vi "Main.vi"(8 "error in":errorcluster, 11 "UserInterface in":refnum<class "UserInterface.lvclass">) -> (0 "error out":errorcluster, 3 "UserInterface out":refnum<class "UserInterface.lvclass">)   [LabVIEW 2021, in "UserInterface.lvclass"]
doc: "The Queued Message Handler of a Worker."
uses:
  UserInterface.lvclass
  C:/Program Files (x86)/National Instruments/LabVIEW 2021/vi.lib/addons/_Workers/Library/Classes/Worker/Worker.lvclass
  <vilib>/addons/_Workers/Library/Classes/Worker/Worker.lvclass/Worker.ctl
  UserInterface.lvclass/UserInterface.ctl
  WaveGenerator/WaveGenerator.lvclass
  Sine/Sine.lvclass
  C:/Users/chrismadlax/Desktop/LVSampleCode/WorkersComposite/Workers/WaveGenerator/WaveGenerator.lvclass
  Square/Square.lvclass
  Triangle/Triangle.lvclass
  <vilib>/addons/_Workers/Library/Classes/Message/Priority.ctl
  <vilib>/addons/_Workers/Library/Classes/Callback Message/Enqueue and Forget.vi
  <vilib>/addons/_Workers/Library/Classes/Message/Enqueue Message to Queue.vi
  <vilib>/addons/_Workers/Library/Classes/Callback Message/Enqueue and Collect.vi
  <vilib>/addons/_Workers/Library/Classes/Message/Enqueue Message to Self v2.vi
  Initialization Data.ctl
  <vilib>/addons/_Workers/Library/Classes/Worker/Worker.lvclass
  <vilib>/addons/_Workers/Library/Classes/Callback Message/Callback Message.lvclass
  <vilib>/addons/_Workers/Library/Classes/Message/Message.lvclass
  C:/Program Files (x86)/National Instruments/LabVIEW 2021/vi.lib/addons/_Workers/Library/Classes/Workers Object/Workers Object.lvclass
  C:/Users/chrismadlax/Desktop/LVSampleCode/WorkersComposite/Workers/UserInterface/UserInterface.lvclass
  <vilib>/addons/_Workers/Library/Classes/Message Queue/Message Queue.lvclass
panel:
  in  "StopM":bool
  out "ID":string
  in  "Destory":bool
  in  "Create":bool
  in  "Text Ring":enum16{"None", "Sine", "Square", "Triangle"}(ring)
  in  "Measure":bool
  out "W.Graph":waveform(dbl)(graph)
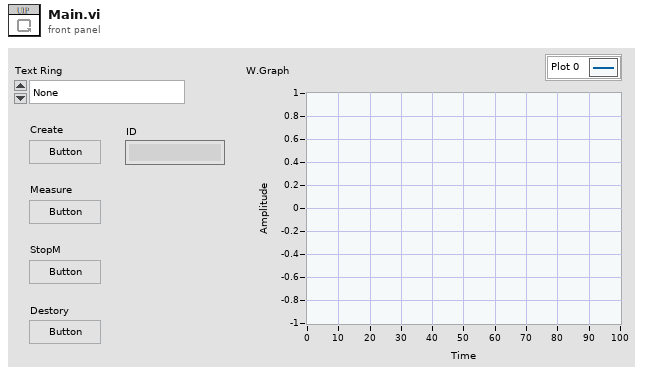
[diagram p1: front panel]
types:
  T1 = typedef "UserInterface.lvclass/Initialization Data.ctl" = cluster{"String":string}
  T2 = typedef "Workers.lvlib/Message.lvclass/Priority.ctl" = enum16{"Low", "Normal", "High"}
  T3 = typedef "Workers.lvlib/Case Label.ctl" = string
  T4 = cluster{"Message Queue out":refnum<class "Message Queue.lvclass">, "Case Label":T3}
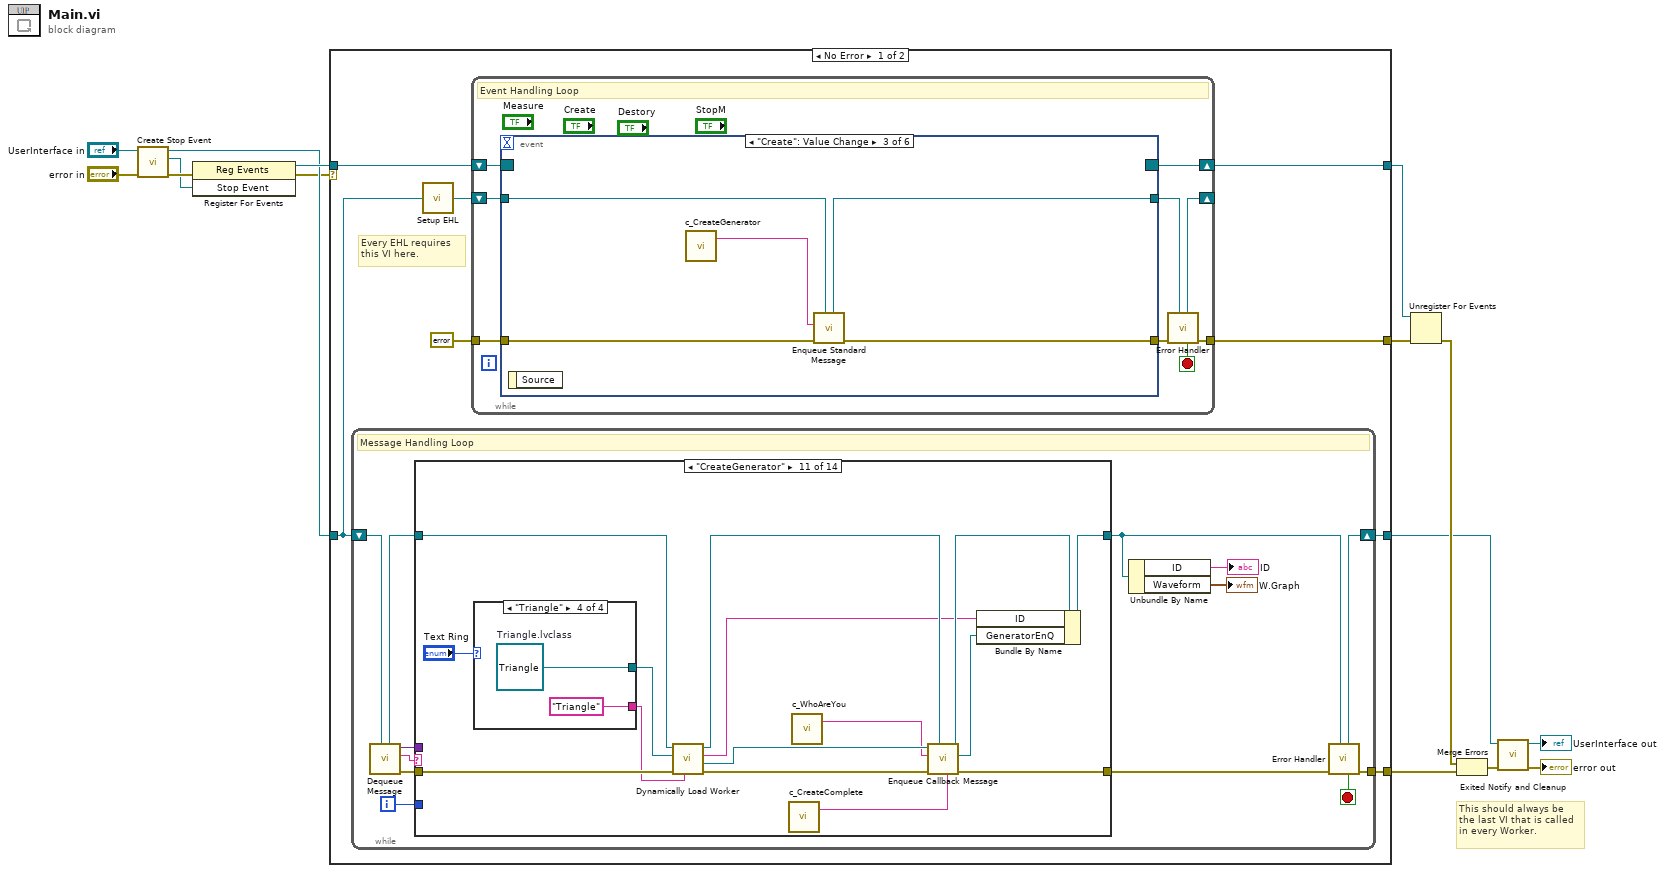
[diagram p0: block diagram]
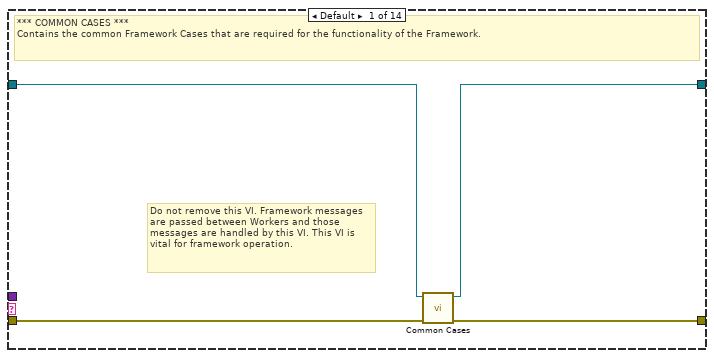
[diagram p2: hidden frame]
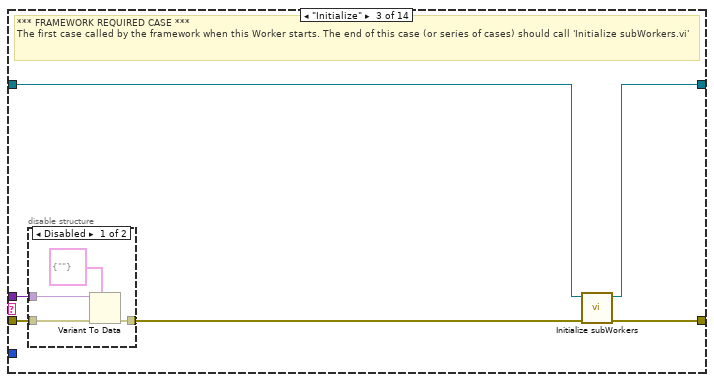
[diagram p4: hidden frame]
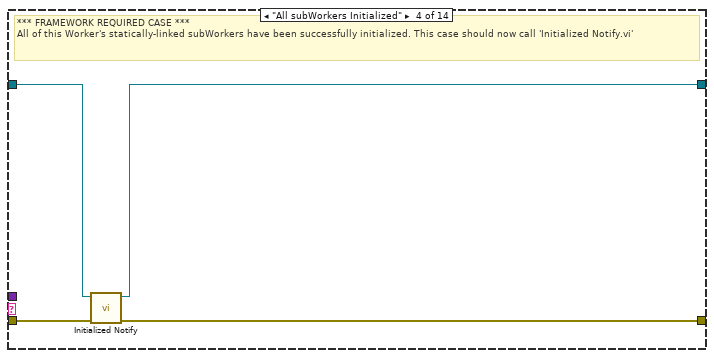
[diagram p6: hidden frame]
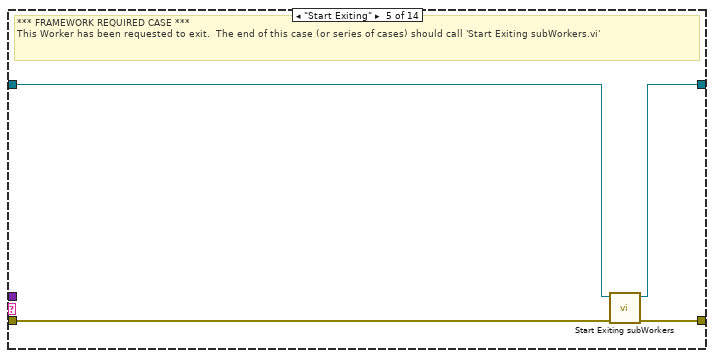
[diagram p7: hidden frame]
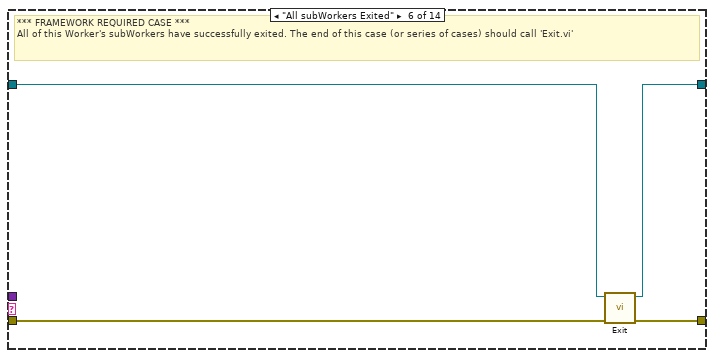
[diagram p8: hidden frame]
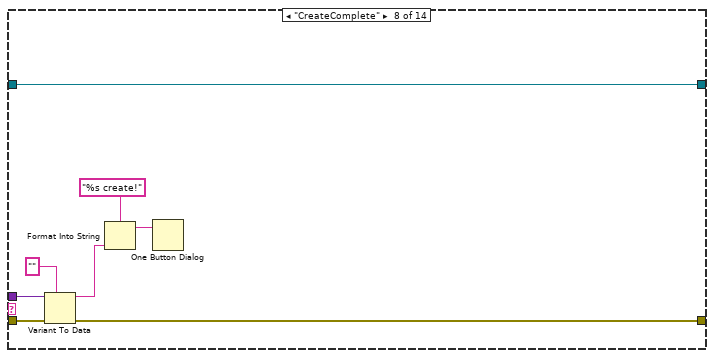
[diagram p10: hidden frame]
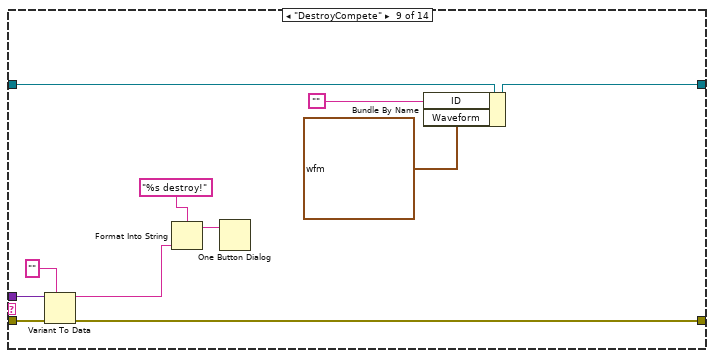
[diagram p11: hidden frame]
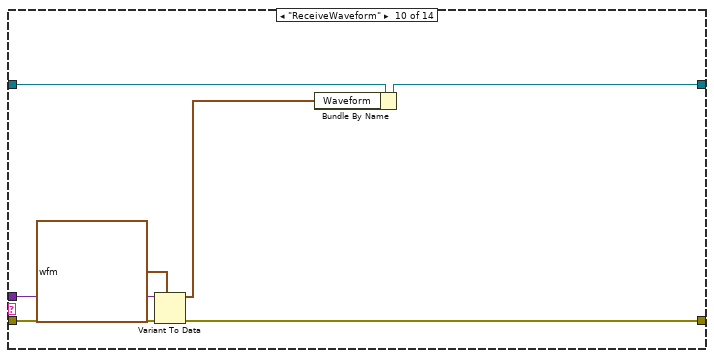
[diagram p12: hidden frame]
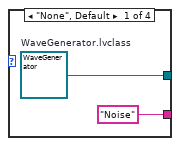
[diagram p13: hidden frame]
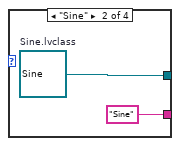
[diagram p14: hidden frame]
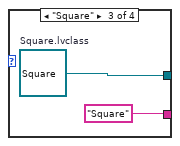
[diagram p15: hidden frame]
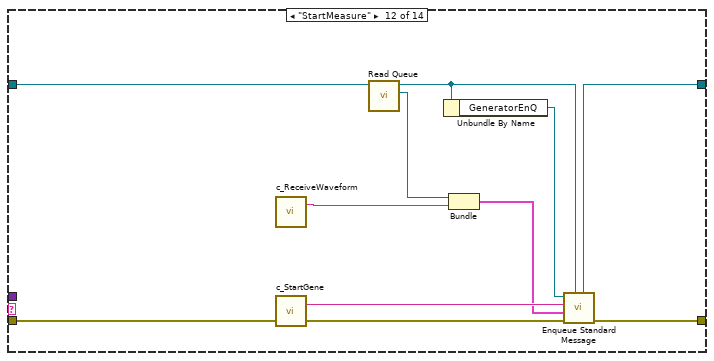
[diagram p16: hidden frame]
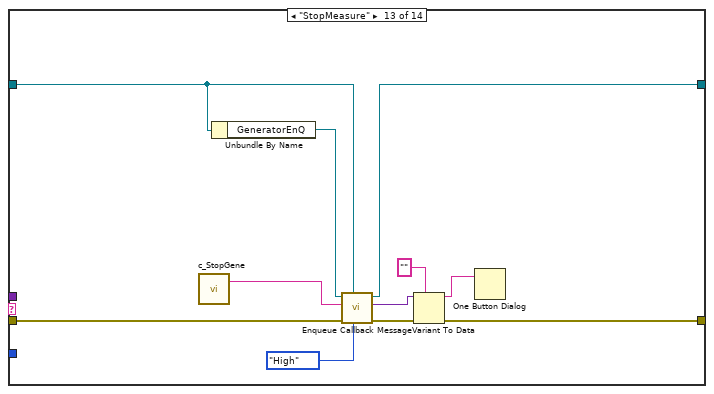
[diagram p17: hidden frame]
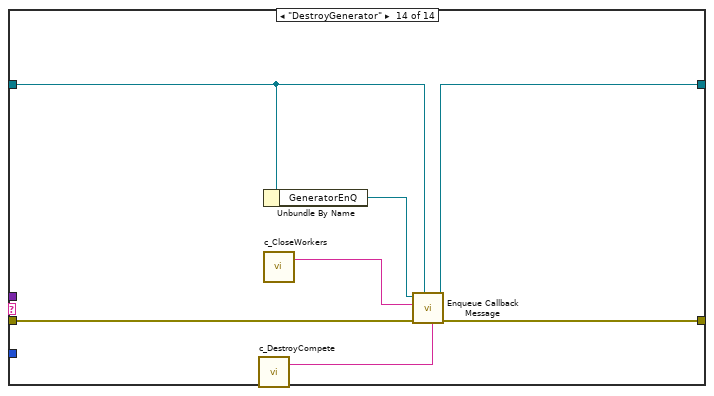
[diagram p18: hidden frame]
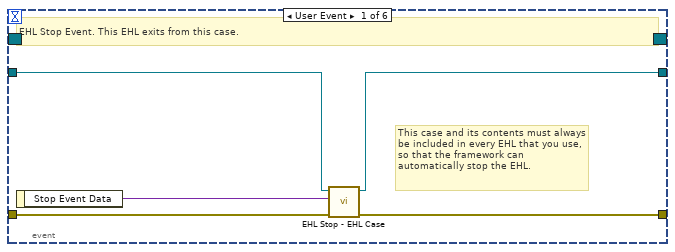
[diagram p19: hidden frame]
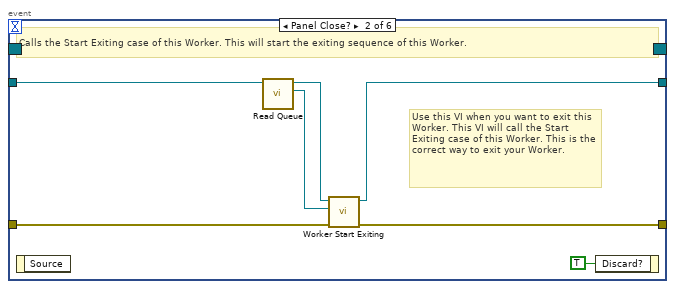
[diagram p20: hidden frame]
diagram:
  # "This should always be the last VI that is called in every Worker."
  n1 = call-dynamic "Create Stop Event.vi"("error in"="error in", "Worker"="UserInterface in") -> ("error out"=w10:errorcluster, "Stop Event"=w7:refnum<user-event>, "Worker out"=w4:refnum<class "UserInterface.lvclass">)  [unwired: 7 in]
  n2 = register-events(error in=w10, w7) -> (reference out=w9:refnum<event-registration>, error out=w2:errorcluster)  [unwired: 1 in]
  n3 = case shown="No Error" w2 {
    tunnel: w4 -> [w18 w187]
    tunnel: [w16 w188] -> w8
    tunnel: w9 -> [w23 w189]
    tunnel: [w20 w190] -> w14
    tunnel: [w22 w189] -> w13
    tunnel: [w17 w186] -> w11
    selector: w2 -> [_ w190]
    frame No Error {
      # "Every EHL requires\nthis VI here."
      n4 = while {
        shift-right: [w34] -> w17
        shift-left: w18 -> [w36]
        tunnel: [w35] -> w16
        i -> [w27]
        stop <- w28 stop-if-true
        # "Message Handling Loop"
        n5 = call-dynamic "Dequeue Message.vi"("Worker"=w36) -> ("error out"=w33:errorcluster, "Case out"=w29:string, "Data out"=w30:variant, "Worker out"=w31:refnum<class "UserInterface.lvclass">)  [unwired: 6 in, 1 out]
        n6 = case "Worker MHL Case Structure (DO NOT CHANGE LABEL NAME)" shown="\"CreateGenerator\"" w29 {
          tunnel: w33 -> [w40 w41 w46 w55 w58 w65 w66 w75 w86 w93 w108 w126 w137 w144]
          tunnel: [w39 w41 w48 w54 w61 w64 w66 w73 w84 w91 w101 w123 w130 w143] -> w32
          tunnel: w31 -> [w38 w42 w43 w57 w59 w63 w67 w74 w85 w92 w106 w125 w134 w141]
          tunnel: [w37 w42 w47 w56 w60 w62 w67 w74 w78 w88 w102 w122 w135 w142] -> w26
          tunnel: w30 -> [_ _ w44 _ _ _ _ w72 w83 w89 _ _ _ _]
          tunnel: w27 -> [_ _ _ _ _ _ _ _ _ _ _ _ _ _]
          frame Default {
            # "Do not remove this VI. Framework messages are passed between Workers and those messages are handled by this VI. This VI is vital for framework operation."
            # "*** COMMON CASES ***\nContains the common Framework Cases that are required for the functionality of the Framework."
            n7 = call-dynamic "Common Cases.vi"("error in"=w40, "Worker in"=w38) -> ("error out"=w39:errorcluster, "Worker out"=w37:refnum<class "UserInterface.lvclass">)  [unwired: 8 in]
          }
          frame "------ FRAMEWORK REQUIRED CASES ------" {
            # "Start of Framework Required Cases"
          }
          frame "Initialize" {
            # "*** FRAMEWORK REQUIRED CASE ***\nThe first case called by the framework when this Worker starts. The end of this case (or series of cases) should call 'Initialize subWorkers.vi'"
            n8 = disable-structure shown="Disabled" {
              disable-tunnel: w46 -> [w52 w53]
              disable-tunnel: [w51 w53] -> w45
              disable-tunnel: w44 -> [w50 _]
              frame Disabled {
                n9 = Variant To Data(error in=w52, type=T1 {"String"=""} ("Initialization Data"), Variant=w50) -> (error out=w51:errorcluster)  [unwired: 1 out]
              }
              frame Enabled {
              }
            }
            n10 = call-dynamic "Initialize subWorkers.vi"("error in"=w45, "Worker"=w43) -> ("error out"=w48:errorcluster, "dup Worker out"=w47:refnum<class "UserInterface.lvclass">)  [unwired: 8 in]
          }
          frame "All subWorkers Initialized" {
            # "*** FRAMEWORK REQUIRED CASE ***\nAll of this Worker's statically-linked subWorkers have been successfully initialized. This case should now call 'Initialized Notify.vi'"
            n11 = call-dynamic "Initialized Notify.vi"("error in"=w55, "Worker"=w57) -> ("error out"=w54:errorcluster, "dup Worker out"=w56:refnum<class "UserInterface.lvclass">)  [unwired: 8 in]
          }
          frame "Start Exiting" {
            # "*** FRAMEWORK REQUIRED CASE ***\nThis Worker has been requested to exit.  The end of this case (or series of cases) should call 'Start Exiting subWorkers.vi'"
            n12 = call-dynamic "Start Exiting subWorkers.vi"("error_in"=w58, "Worker"=w59) -> ("error out"=w61:errorcluster, "dup Worker out"=w60:refnum<class "UserInterface.lvclass">)  [unwired: 8 in]
          }
          frame "All subWorkers Exited" {
            # "*** FRAMEWORK REQUIRED CASE ***\nAll of this Worker's subWorkers have successfully exited. The end of this case (or series of cases) should call 'Exit.vi'"
            n13 = call-dynamic "Exit.vi"("error_in"=w65, "Worker"=w63) -> ("error out"=w64:errorcluster, "dup Worker out"=w62:refnum<class "UserInterface.lvclass">)  [unwired: 8 in]
          }
          frame "-----------------------------------------------" {
            # "End of Framework Required Cases"
          }
          frame "CreateComplete" {
            n14 = Variant To Data(error in=w75, type="", Variant=w72) -> (data=w69:string, error out=w73:errorcluster)
            n15 = Format Into String(format string="%s create!", w69) -> (resulting string=w68:string)  [unwired: 2 in, 1 out]
            n16 = One Button Dialog(message=w68) -> ()  [unwired: 1 in, 1 out]
          }
          frame "DestroyCompete" {
            n17 = Variant To Data(error in=w86, type="", Variant=w83) -> (data=w80:string, error out=w84:errorcluster)
            n18 = Format Into String(format string="%s destroy!", w80) -> (resulting string=w79:string)  [unwired: 2 in, 1 out]
            n19 = One Button Dialog(message=w79) -> ()  [unwired: 1 in, 1 out]
            n20 = Bundle By Name(cluster=w85, "ID"="", "Waveform"=waveform(dbl) {"t0"=timestamp(0 s since 1904-01-01), "dt"=1.0, "Y"=[]}) -> (w78:refnum<class "UserInterface.lvclass">)
          }
          frame "ReceiveWaveform" {
            n21 = Variant To Data(error in=w93, type=waveform(dbl) {"t0"=timestamp(0 s since 1904-01-01), "dt"=1.0, "Y"=[]} ("Waveform"), Variant=w89) -> (data=w87:waveform(dbl), error out=w91:errorcluster)
            n22 = Bundle By Name(cluster=w92, "Waveform"=w87) -> (w88:refnum<class "UserInterface.lvclass">)
          }
          frame "CreateGenerator" {
            n23 = case shown="\"Triangle\"" "Text Ring" {
              tunnel: [w110 w112 w114 w115] -> w104
              tunnel: ["Noise" ("Worker Alias") "Sine" ("Worker Alias") "Square" ("Worker Alias") "Triangle" ("Worker Alias")] -> w103
              frame "None", Default {
                w110 = refnum<class "WaveGenerator.lvclass"> refnum  # WaveGenerator.lvclass
              }
              frame "Sine" {
                w112 = refnum<class "Sine.lvclass"> refnum  # Sine.lvclass
              }
              frame "Square" {
                w114 = refnum<class "Square.lvclass"> refnum  # Square.lvclass
              }
              frame "Triangle" {
                w115 = refnum<class "Triangle.lvclass"> refnum  # Triangle.lvclass
              }
            }
            n24 = call <vilib>:"Dynamically Load Worker.vi"("Worker Alias"=w103, "error in"=w108, "Worker to Dynamically Load"=w104, "Worker"=w106) -> ("error out"=w107:errorcluster, "Message Queue out"=w98:refnum<class "Message Queue.lvclass">, "ID out"=w94:string, "dup Worker out"=w100:refnum<class "UserInterface.lvclass">)  [unwired: 4 in]
            n25 = call "c_CreateComplete.vi"() -> ("Case Label"=w95:T3)  [unwired: 1 in]
            n26 = call "c_WhoAreYou.vi"() -> ("Case Label"=w96:T3)  [unwired: 1 in]
            n27 = call-poly <vilib>:"Enqueue Callback Message.vi"("Callback Case Label"=w95, "Worker"=w100, "error in"=w107, "Case Label"=w96, "Message Queue"=w98) -> ("error out"=w101:errorcluster, "dup Message Queue out"=w97:refnum<class "Message Queue.lvclass">, "dup Worker out"=w99:refnum<class "UserInterface.lvclass">)  [unwired: 4 in]
            n28 = Bundle By Name(cluster=w99, "ID"=w94, "GeneratorEnQ"=w97) -> (w102:refnum<class "UserInterface.lvclass">)
          }
          frame "StartMeasure" {
            n29 = call "c_ReceiveWaveform.vi"() -> ("Case Label"=w119:T3)  [unwired: 1 in]
            n30 = call "c_StartGene.vi"() -> ("Case Label"=w118:T3)  [unwired: 1 in]
            n31 = call <vilib>:"Read Queue.vi"("Worker"=w125) -> ("Message Queue out"=w120:refnum<class "Message Queue.lvclass">, "dup Worker out"=w121:refnum<class "UserInterface.lvclass">)  [unwired: 9 in]
            n32 = Unbundle By Name(w121) -> ("GeneratorEnQ"=w124:refnum<class "Message Queue.lvclass">)
            n33 = Bundle("Message Queue out"=w120, "Case Label"=w119) -> (w117:T4)  [unwired: 1 in]
            n34 = call-poly <vilib>:"Enqueue Standard Message.vi"("Worker"=w121, "error in"=w126, "Data"=w117, "Case Label"=w118, "Message Queue"=w124) -> ("error out"=w123:errorcluster, "dup Worker out"=w122:refnum<class "UserInterface.lvclass">)  [unwired: 4 in, 1 out]
          }
          frame "StopMeasure" {
            n35 = call "c_StopGene.vi"() -> ("Case Label"=w132:T3)  [unwired: 1 in]
            n36 = Unbundle By Name(w134) -> ("GeneratorEnQ"=w133:refnum<class "Message Queue.lvclass">)
            n37 = call-poly <vilib>:"Enqueue Callback Message.vi"("Priority (Normal)"=Priority."High", "Worker"=w134, "error in"=w137, "Case Label"=w132, "Message Queue"=w133) -> ("error out"=w136:errorcluster, "Data out"=w129:variant, "dup Worker out"=w135:refnum<class "UserInterface.lvclass">)  [unwired: 3 in, 1 out]
            n38 = Variant To Data(error in=w136, type="", Variant=w129) -> (data=w127:string, error out=w130:errorcluster)
            n39 = One Button Dialog(message=w127) -> ()  [unwired: 1 in, 1 out]
          }
          frame "DestroyGenerator" {
            n40 = call "c_DestroyCompete.vi"() -> ("Case Label"=w138:T3)  [unwired: 1 in]
            n41 = Unbundle By Name(w141) -> ("GeneratorEnQ"=w140:refnum<class "Message Queue.lvclass">)
            n42 = call "c_CloseWorkers.vi"() -> ("Case Label"=w139:T3)  [unwired: 1 in]
            n43 = call-poly <vilib>:"Enqueue Callback Message.vi"("Callback Case Label"=w138, "Worker"=w141, "error in"=w144, "Case Label"=w139, "Message Queue"=w140) -> ("error out"=w143:errorcluster, "dup Worker out"=w142:refnum<class "UserInterface.lvclass">)  [unwired: 4 in, 1 out]
          }
        }
        n44 = Unbundle By Name(w26) -> ("ID"=→"ID":string, "Waveform"=→"W.Graph":waveform(dbl))
        n45 = call-dynamic "Error Handler.vi"("Worker"=w26, "error_in"=w32) -> ("error out"=w35:errorcluster, "Stop Loop"=w28:bool, "Worker out"=w34:refnum<class "UserInterface.lvclass">)  [unwired: 7 in]
      }
      n46 = call-dynamic "Setup EHL.vi"("Worker"=w18) -> ("Worker out"=w19:refnum<class "UserInterface.lvclass">)  [unwired: 14 in]
      n47 = while "Event Handling Loop" {
        shift-right: [w153] -> w22
        shift-left: w23 -> [w152]
        tunnel: [w148] -> w20
        tunnel: errorcluster {"status"=FALSE, "code"=0, "source"=""} ("error constant") -> [w150]
        shift-right: [w146] -> _
        shift-left: w19 -> [w151]
        stop <- w145 stop-if-true
        # "Event Handling Loop"
        n48 = event shown="[2] \"Create\": Value Change" {
          selector: w152 -> [_ _ _ _ _ _]
          dyn-events: [_ _ _ _ _ _] -> w153
          timeout: _ -> [_ _ _ _ _ _]
          tunnel: [w157 w164 w169 w174 w179 w184] -> w149
          tunnel: w150 -> [w158 w163 w170 w175 w180 w185]
          tunnel: w151 -> [w156 w162 w168 w173 w178 w183]
          tunnel: [w155 w161 w167 w172 w177 w182] -> w147
          event User Event {
            # "This case and its contents must always be included in every EHL that you use, so that the framework can automatically stop the EHL."
            # "EHL Stop Event. This EHL exits from this case."
            n49 = event-data() -> ("Stop Event Data"=w154:variant)  [unwired: 1 in]
            n50 = call <vilib>:"EHL Stop - EHL Case.vi"("error in"=w158, "Stop Event Data"=w154, "Worker"=w156) -> ("error out"=w157:errorcluster, "Worker out"=w155:refnum<class "UserInterface.lvclass">)  [unwired: 7 in]
          }
          event Panel Close? {
            # "Use this VI when you want to exit this Worker. This VI will call the Start Exiting case of this Worker. This is the correct way to exit your Worker."
            # "Calls the Start Exiting case of this Worker. This will start the exiting sequence of this Worker."
            n51 = event-data() -> ()  [unwired: 1 in, 1 out]
            n52 = call <vilib>:"Read Queue.vi"("Worker"=w162) -> ("Message Queue out"=w159:refnum<class "Message Queue.lvclass">, "dup Worker out"=w160:refnum<class "UserInterface.lvclass">)  [unwired: 9 in]
            n53 = call-dynamic "Worker Start Exiting.vi"("error_in"=w163, "Message Queue"=w159, "Worker"=w160) -> ("error out"=w164:errorcluster, "dup Worker out"=w161:refnum<class "UserInterface.lvclass">)  [unwired: 7 in]
            n54 = event-data ("Event Filter Node")("Discard?"=TRUE) -> ()  [unwired: 1 in, 1 out]
          }
          event "Create": Value Change {
            n55 = event-data() -> ()  [unwired: 1 in, 1 out]
            n56 = call "c_CreateGenerator.vi"() -> ("Case Label"=w166:T3)  [unwired: 1 in]
            n57 = call-poly <vilib>:"Enqueue Standard Message.vi"("Worker"=w168, "error in"=w170, "Case Label"=w166) -> ("error out"=w169:errorcluster, "dup Worker out"=w167:refnum<class "UserInterface.lvclass">)  [unwired: 7 in]
          }
          event "Measure": Value Change {
            n58 = event-data() -> ()  [unwired: 1 in, 1 out]
            n59 = call "c_StartMeasure.vi"() -> ("Case Label"=w171:T3)  [unwired: 1 in]
            n60 = call-poly <vilib>:"Enqueue Standard Message.vi"("Worker"=w173, "error in"=w175, "Case Label"=w171) -> ("error out"=w174:errorcluster, "dup Worker out"=w172:refnum<class "UserInterface.lvclass">)  [unwired: 7 in]
          }
          event "StopM": Value Change {
            n61 = event-data() -> ()  [unwired: 1 in, 1 out]
            n62 = call "c_StopMeasure.vi"() -> ("Case Label"=w176:T3)  [unwired: 1 in]
            n63 = call-poly <vilib>:"Enqueue Standard Message.vi"("Worker"=w178, "error in"=w180, "Case Label"=w176) -> ("error out"=w179:errorcluster, "dup Worker out"=w177:refnum<class "UserInterface.lvclass">)  [unwired: 7 in]
          }
          event "Destory": Value Change {
            n64 = event-data() -> ()  [unwired: 1 in, 1 out]
            n65 = call "c_DestroyGenerator.vi"() -> ("Case Label"=w181:T3)  [unwired: 1 in]
            n66 = call-poly <vilib>:"Enqueue Standard Message.vi"("Worker"=w183, "error in"=w185, "Case Label"=w181) -> ("error out"=w184:errorcluster, "dup Worker out"=w182:refnum<class "UserInterface.lvclass">)  [unwired: 7 in]
          }
        }
        n67 = call-dynamic "Error Handler.vi"("Worker"=w147, "error_in"=w149) -> ("error out"=w148:errorcluster, "Stop Loop"=w145:bool, "Worker out"=w146:refnum<class "UserInterface.lvclass">)  [unwired: 7 in]
      }
    }
    frame Error {
      n68 = call-dynamic "Error Handler.vi"("Worker"=w187, "error_in"=w190) -> ("error out"=w188:errorcluster, "Worker out"=w186:refnum<class "UserInterface.lvclass">)  [unwired: 7 in, 1 out]
    }
  }
  n69 = Unregister For Events(event registration refnum=w13, error in=w14) -> (error out=w15:errorcluster)
  n70 = Merge Errors(w15, w8) -> (w12:errorcluster)
  n71 = call-dynamic "Exited Notify and Cleanup.vi"("error_in"=w12, "Worker"=w11) -> ("error out"=→"error out":errorcluster, "dup Worker out"=→"UserInterface out":refnum<class "UserInterface.lvclass">)  [unwired: 8 in]
